vi "CreateScanPattern.vi"(6 "AO\nrow: rest, illumination\ncol: X, Y, Z":dbl[][](array[numeric])=[[5.0, 5.0, 0.0, 0.0, 0.0, 1.0], [-0.2, 2.9, 0.0, 0.0, 0.0, 0.0]], 8 "Timing":T2={"Size (pix)"=1024, "Exposure (s)"=0.1, "Slice (s)"=0.0, "Series (s)"=0.0} {"Size (pix)" items=["2048"=2048, "1024"=1024, "512"=512, "256"=256]}, 9 "Beam":T5={"n spirals"=5, "A spiral (V)"=0.8, "sigma"=2.0, "SLIM"=TRUE}, 10 "DAQ":T4={"Ramp time (s)"=0.01, "DAQ rate (Hz)"=10000.0, "X0 (V)"=5.0, "Xc (V)"=-0.2, "Y0 (V)"=5.0, "Yc (V)"=-0.2, "Z0 (V)"=0.0, "Zc (V)"=0.0}, 11 "Stack":T3={"LED (V)"=1.0, "#z steps"=1, "z step (V)"=1.0, "UV (%)"=0.2} {"UV (%)" format="%#_13g"}) -> (1 "AO (V)":dbl[][](array[numeric]), 3 "Camera \nExposure Time (ms)":dbl=17.0, 4 "DO":digitaldata[](array[digital]), 5 "All signals":dbl[][](graph))   [LabVIEW 2018]
uses:
  <vilib>/Analysis/1siggen.llb/Ramp Pattern by Samples.vi
  <vilib>/Analysis/baseanly.llb/Mean (DBL).vi
  <vilib>/Analysis/NI_AALBase.lvlib
panel:
  in  "45 Degrees":bool
  in  "A_y":dbl=0.86 format="%#_13g"
  in  "Additional Sweeps/Line":u32=3
  out "fraction exposed":dbl=0.89
  out "Camera\nreadout time (ms)":u64=11
  in  "Channels":T1(ring)=enum."UV"
  out "error out (no error)":errorcluster
  in  "error in (no error)":errorcluster
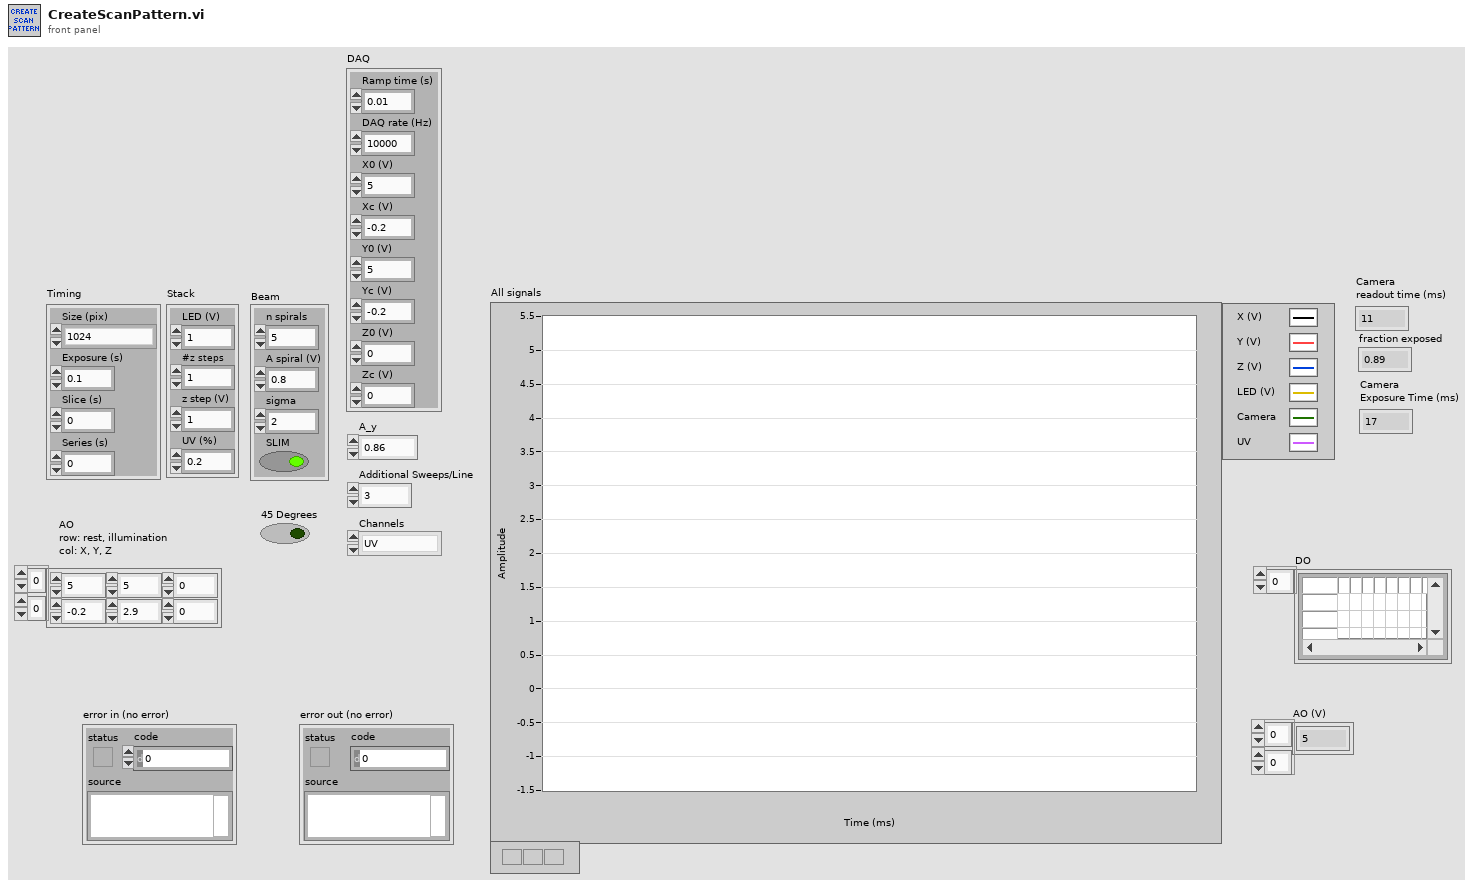
[diagram p1: front panel]
types:
  T1 = enum16{"X (V)", "Y (V)", "Z (V)", "LED (V)", "Camera", "UV"}
  T2 = cluster{"Size (pix)":u16, "Exposure (s)":dbl, "Slice (s)":dbl, "Series (s)":dbl}
  T3 = cluster{"LED (V)":dbl, "#z steps":i64, "z step (V)":dbl, "UV (%)":dbl}
  T4 = cluster{"Ramp time (s)":dbl, "DAQ rate (Hz)":dbl, "X0 (V)":dbl, "Xc (V)":dbl, "Y0 (V)":dbl, "Yc (V)":dbl, "Z0 (V)":dbl, "Zc (V)":dbl}
  T5 = cluster{"n spirals":u32, "A spiral (V)":dbl, "sigma":dbl, "SLIM":bool}
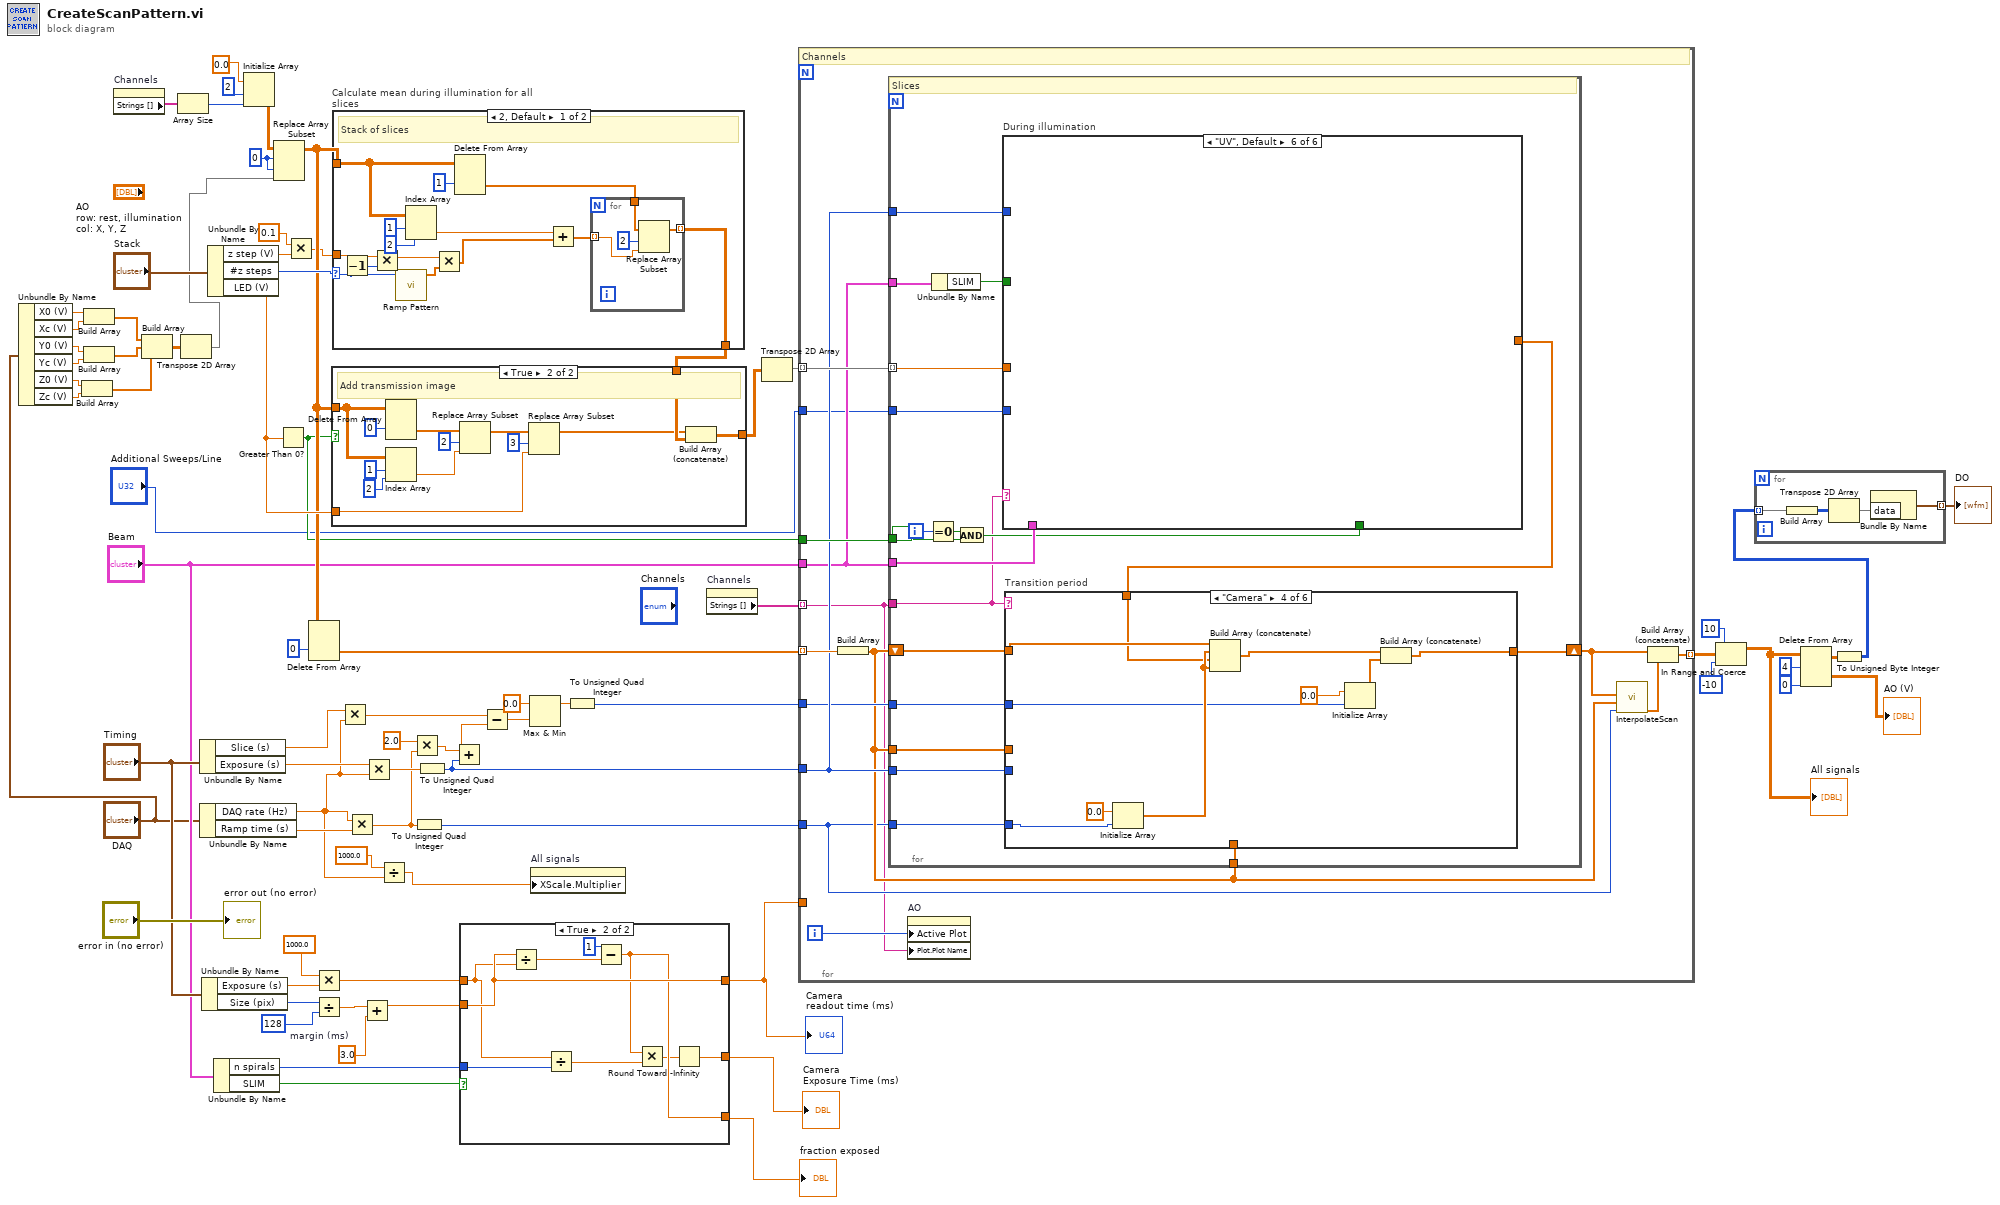
[diagram p0: block diagram]
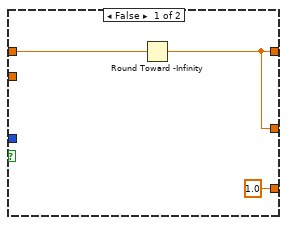
[diagram p2: hidden frame]
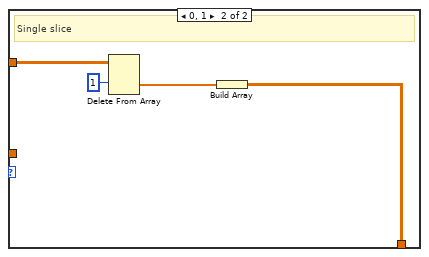
[diagram p4: hidden frame]
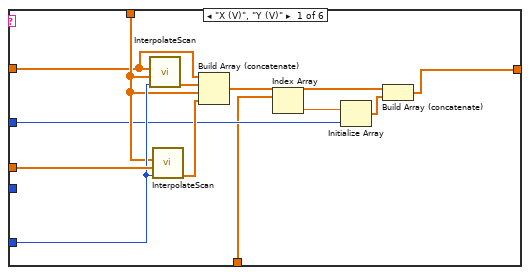
[diagram p5: hidden frame]
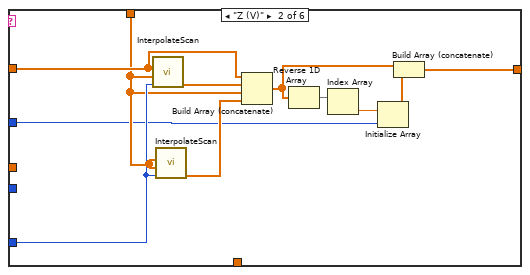
[diagram p6: hidden frame]
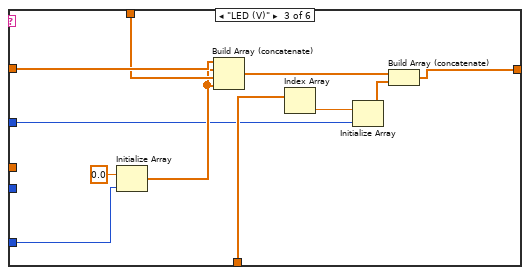
[diagram p7: hidden frame]
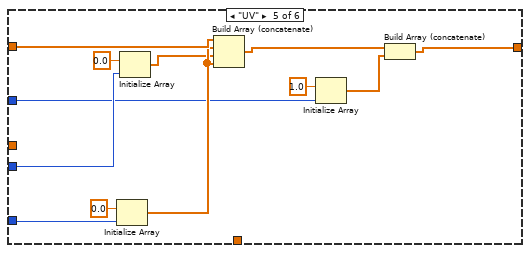
[diagram p8: hidden frame]
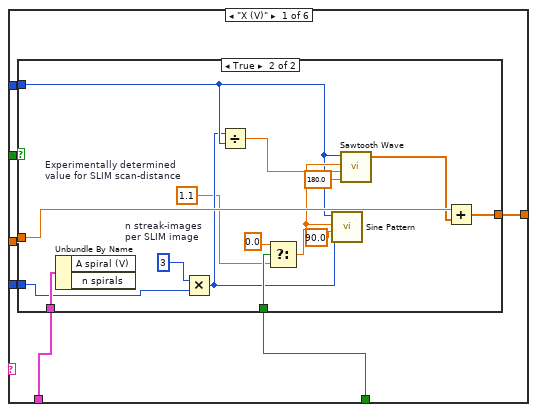
[diagram p10: hidden frame]
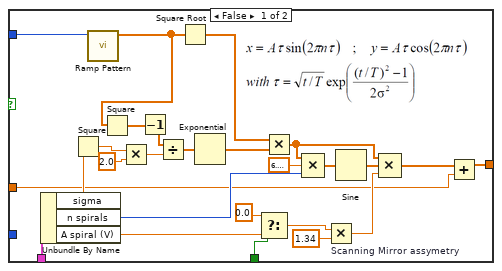
[diagram p11: hidden frame]
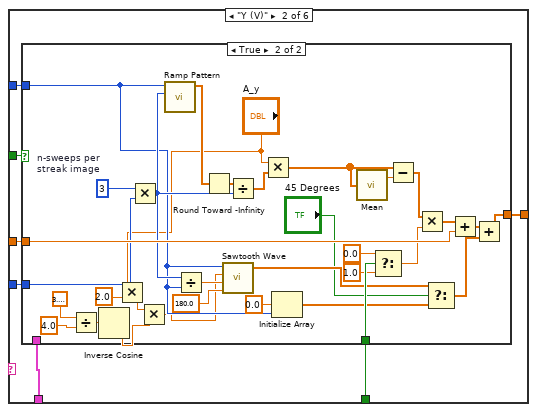
[diagram p12: hidden frame]
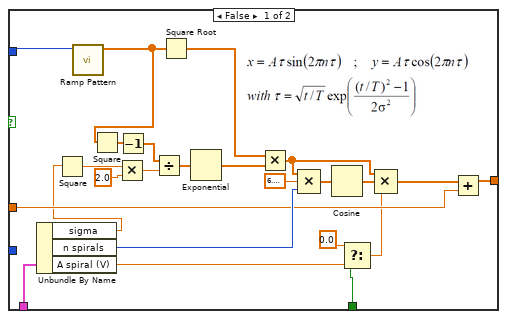
[diagram p13: hidden frame]
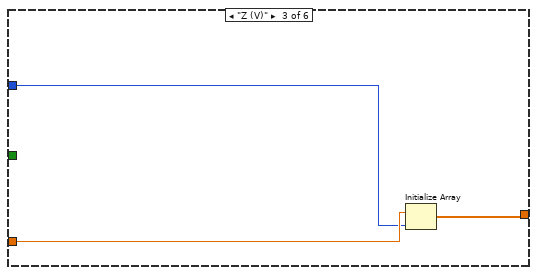
[diagram p14: hidden frame]
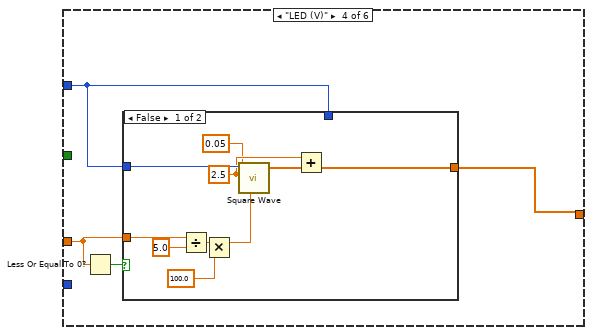
[diagram p15: hidden frame]
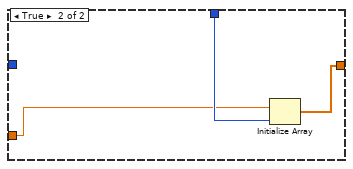
[diagram p16: hidden frame]
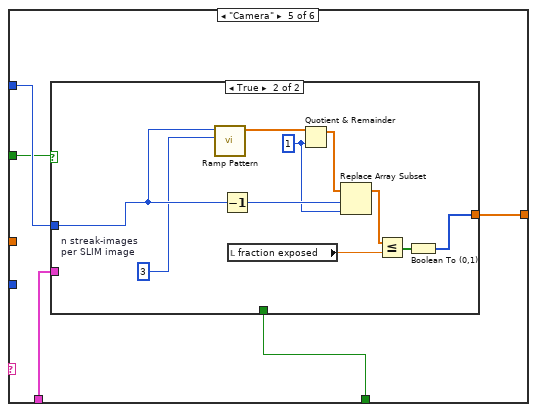
[diagram p17: hidden frame]
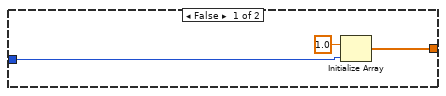
[diagram p18: hidden frame]
diagram:
  w27 = 3.0  # margin (ms)
  w63 = 0 ("index (row)")
  n1 = Unbundle By Name("DAQ") -> ("X0 (V)"=w11:dbl, "Xc (V)"=w10:dbl, "Y0 (V)"=w9:dbl, "Yc (V)"=w8:dbl, "Z0 (V)"=w6:dbl, "Zc (V)"=w7:dbl)
  n2 = Build Array(w6, w7) -> (w3:dbl[])
  n3 = Build Array(w11, w10) -> (w5:dbl[])
  n4 = Build Array(w9, w8) -> (w4:dbl[])
  n5 = property on="Channels" class="Enum (strict)"() -> ("Strings []"=w54:string[])  [unwired: 2 in, 2 out]
  n6 = Build Array(w5, w4, w3) -> (w2:dbl[][])
  n7 = Array Size(array=w54) -> (size(s)=w53:i32)
  n8 = Transpose 2D Array(2D array=w2) -> (transposed array=w1:dbl[][])
  n9 = Unbundle By Name("Timing") -> ("Slice (s)"=w61:dbl, "Exposure (s)"=w77:dbl)
  n10 = Unbundle By Name("DAQ") -> ("DAQ rate (Hz)"=w32:dbl, "Ramp time (s)"=w71:dbl)
  n11 = Unbundle By Name("Timing") -> ("Exposure (s)"=w34:dbl, "Size (pix)"=w40:u16)
  n12 = Unbundle By Name("Stack") -> ("z step (V)"=w17:dbl, "#z steps"=w72:i64, "LED (V)"=w68:dbl)
  n13 = Unbundle By Name("Beam") -> ("n spirals"=w36:u32, "SLIM"=w38:bool)
  n14 = Initialize Array(0.0 ("dimension size"), 2 ("dimension size"), w53) -> (w64:dbl[][])
  n15 = Replace Array Subset(array=w64, new element=w1, index (row)=w63, index (col)=w63) -> (w62:dbl[][])
  n16 = Greater Than 0?(x=w68) -> (x > 0?=w52:bool)
  n17 = Multiply(x=0.1, y=w17) -> (x*y=w18:dbl)
  n18 = Delete From Array(array=w62, index (row)=0) -> (deleted portion=w13:dbl[])  [unwired: 2 in, 1 out]
  n19 = Multiply(x=1000.0 ("y"), y=w34) -> (x*y=w33:dbl)
  n20 = Divide(x=w40, y=u16 128) -> (x/y=w37:dbl)
  n21 = case "Calculate mean during illumination for all slices" shown="2, Default" w72 {
    selector: w72 -> [w80 _]
    tunnel: w62 -> [w84 w98]
    tunnel: w18 -> [w90 _]
    tunnel: [w83 w97] -> w70
    frame 2, Default {
      # "Stack of slices"
      n22 = Decrement(x=w80) -> (x-1=w79:i64)
      n23 = Multiply(x=w90, y=w79) -> (x*y=w81:dbl)
      n24 = call-poly <vilib>:"Ramp Pattern.vi"("samples"=w80) -> ("Ramp Pattern"=w91:dbl[])  [unwired: 9 in, 1 out]
      n25 = Index Array(array=w84, index (row)=1, index (col)=2 ("disabled index (col)")) -> (element=w87:dbl)
      n26 = Multiply(x=w81, y=w91) -> (x*y=w78:dbl[])
      n27 = Delete From Array(array=w84, index (row)=1) -> (deleted portion=w82:dbl[])  [unwired: 2 in, 1 out]
      n28 = Add(x=w87, y=w78) -> (x+y=w86:dbl[])
      n29 = for {
        tunnel: w86 -> [w93] mode=indexing
        tunnel: w82 -> [w95]
        tunnel: [w92] -> w83 mode=indexing
        n30 = Replace Array Subset(array=w95, new element=w93, index=2) -> (w92:dbl[])
      }
    }
    frame 0, 1 {
      # "Single slice"
      n31 = Delete From Array(array=w98, index (row)=1) -> (deleted portion=w96:dbl[])  [unwired: 2 in, 1 out]
      n32 = Build Array(w96) -> (w97:dbl[][])
    }
  }
  n33 = case shown="True" w52 {
    tunnel: [w100 w105] -> w69
    tunnel: w70 -> [w100 w106]
    tunnel: w62 -> [_ w110]
    tunnel: w68 -> [_ w101]
    frame False {
      # "No transmission image"
    }
    frame True {
      # "Add transmission image"
      n34 = Delete From Array(array=w110, index (row)=0) -> (deleted portion=w112:dbl[])  [unwired: 2 in, 1 out]
      n35 = Index Array(array=w110, index (row)=1, index (col)=2 ("disabled index (col)")) -> (element=w107:dbl)
      n36 = Replace Array Subset(array=w112, new element=w107, index=2) -> (w103:dbl[])
      n37 = Replace Array Subset(array=w103, new element=w101, index=3) -> (w104:dbl[])
      n38 = Build Array (concatenate)(w104, w106) -> (w105:dbl[][])
    }
  }
  n39 = Multiply(x=w61, y=w32) -> (x*y=w56:dbl)
  n40 = Multiply(x=w32, y=w71) -> (x*y=w60:dbl)
  n41 = Add(x=w37, y=w27) -> (x+y=w28:dbl)
  n42 = Multiply(x=w77, y=w32) -> (x*y=w73:dbl)
  n43 = Divide(x=1000.0, y=w32) -> (x/y=w29:dbl)
  n44 = Multiply(x=2.0, y=w60) -> (x*y=w58:dbl)
  n45 = To Unsigned Quad Integer(1:w60) -> (0:w50:u64)
  n46 = To Unsigned Quad Integer(1:w73) -> (0:w48:u64)
  n47 = Add(x=w58, y=w48) -> (x+y=w57:dbl)
  n48 = case shown="True" w38 {
    tunnel: w28 -> [_ w123]
    tunnel: w36 -> [_ w121]
    tunnel: [w114 w123] -> w15
    tunnel: w33 -> [w115 w122]
    tunnel: [1.0 w119] -> w30
    tunnel: [w114 w117] -> w19
    frame False {
      n49 = Round Toward -Infinity(1:w115) -> (0:w114:dbl)
    }
    frame True {
      n50 = Divide(x=w123, y=w122) -> (x/y=w125:dbl)
      n51 = Divide(x=w122, y=w121) -> (x/y=w120:dbl)
      n52 = Subtract(x=1 ("index (row)"), y=w125) -> (x-y=w119:dbl)
      n53 = Multiply(x=w119, y=w120) -> (x*y=w118:dbl)
      n54 = Round Toward -Infinity(1:w118) -> (0:w117:dbl)
    }
  }
  "Camera\nreadout time (ms)" <- w15
  "fraction exposed" <- w30
  "Camera \nExposure Time (ms)" <- w19
  n55 = Subtract(x=w56, y=w57) -> (x-y=w55:dbl)
  n56 = Max & Min(x=0.0, y=w55) -> (max(x,y)=w47:dbl)  [unwired: 1 out]
  n57 = property on="All signals" class="WFGraph (strict)"("XScale.Multiplier"=w29) -> ()  [unwired: 2 in, 2 out]
  n58 = To Unsigned Quad Integer(1:w47) -> (0:w49:u64)
  n59 = property on="Channels" class="Enum (strict)"() -> ("Strings []"=w75:string[])  [unwired: 2 in, 2 out]
  n60 = Transpose 2D Array(2D array=w69) -> (transposed array=w51:dbl[][])
  n61 = for {
    tunnel: w75 -> [w129] mode=indexing
    tunnel: "Beam" -> [w128]
    tunnel: w51 -> [w139] mode=indexing
    tunnel: w13 -> [w137] mode=indexing
    tunnel: w50 -> [w131]
    tunnel: w49 -> [w133]
    tunnel: w52 -> [w138]
    tunnel: w48 -> [w134]
    tunnel: [w127] -> w24 mode=indexing
    tunnel: w15 -> [_]
    tunnel: "Additional Sweeps/Line" -> [w126]
    i -> [w130]
    # "Channels"
    n62 = Build Array(w137) -> (w132:dbl[])
    n63 = for {
      tunnel: w129 -> [w150]
      tunnel: w128 -> [w158]
      tunnel: w139 -> [w157] mode=indexing
      tunnel: w138 -> [w154]
      tunnel: w134 -> [w152]
      shift-right: [w147] -> w135
      shift-left: w132 -> [w149]
      tunnel: w131 -> [w148]
      tunnel: w132 -> [w146]
      tunnel: w134 -> [w145]
      tunnel: w133 -> [w144]
      tunnel: w132 -> [w143]
      tunnel: w128 -> [w142]
      tunnel: w126 -> [w140]
      i -> [w156]
      # "Slices"
      n64 = Equal To 0?(x=w156) -> (x = 0?=w155:bool)
      n65 = Unbundle By Name(w142) -> ("SLIM"=w141:bool)
      n66 = And(x=w155, y=w154) -> (x .and. y?=w153:bool)
      n67 = case "During illumination" shown="\"UV\", Default" w150 {
        tunnel: w158 -> [w221 w269 _ _ w348 _]
        tunnel: [w220 w268 w329 w333 w351 _] -> w151
        tunnel: w157 -> [w219 w267 w328 w331 _ _]
        tunnel: w153 -> [w218 w266 _ _ w347 _]
        tunnel: w152 -> [w216 w264 w327 w332 w350 _]
        tunnel: w141 -> [w217 w265 _ _ w349 _]
        tunnel: w140 -> [w215 w263 _ _ _ _]
        frame "X (V)" {
          n68 = case shown="True" w217 {
            tunnel: w221 -> [w233 w262]
            tunnel: [w232 w261] -> w220
            tunnel: w219 -> [w231 w257]
            tunnel: w218 -> [w227 w259]
            tunnel: w216 -> [w224 w253]
            tunnel: w215 -> [_ w256]
            frame False {
              n69 = Unbundle By Name(w233) -> ("sigma"=w236:dbl, "n spirals"=w237:u32, "A spiral (V)"=w229:dbl)
              n70 = Square(x=w236) -> (x^2=w247:dbl)
              n71 = call-poly <vilib>:"Ramp Pattern.vi"("samples"=w224) -> ("Ramp Pattern"=w223:dbl[])  [unwired: 9 in, 1 out]
              n72 = Square(x=w223) -> (x^2=w225:dbl[])
              n73 = Multiply(x=w247, y=2.0) -> (x*y=w245:dbl)
              n74 = Decrement(x=w225) -> (x-1=w226:dbl[])
              n75 = Divide(x=w226, y=w245) -> (x/y=w244:dbl[])
              n76 = Square Root(x=w223) -> (sqrt(x)=w243:dbl[])
              n77 = Exponential(1:w244) -> (0:w242:dbl[])
              n78 = Select(t=0.0 ("f"), s=w227, f=w229) -> (s? t:f=w228:dbl)
              n79 = Multiply(x=w243, y=w242) -> (x*y=w239:dbl[])
              n80 = Compound Arithmetic op=MULTIPLY(w239, 6.283185307179586, w237) -> (w238:dbl[])
              n81 = Multiply "Scanning Mirror assymetry"(x=w228, y=1.34 ("x")) -> (x*y=w234:dbl)
              n82 = Sine(x=w238) -> (sin(x)=w240:dbl[])
              n83 = Compound Arithmetic op=MULTIPLY(w239, w240, w234) -> (w222:dbl[])
              n84 = Add(x=w222, y=w231) -> (x+y=w232:dbl[])
            }
            frame True {
              w248 = u32 3  # n streak-images  per SLIM image
              w249 = 1.1  # Experimentally determined  value for SLIM scan-distance
              n85 = Unbundle By Name(w262) -> ()  [unwired: 2 out]
              n86 = Multiply(x=w248, y=w256) -> (x*y=w252:u32)
              n87 = Divide(x=w252, y=w253) -> (x/y=w251:dbl)
              n88 = Select(t=0.0 ("f"), s=w259, f=w249) -> (s? t:f=w255:dbl)
              n89 = call <vilib>:"Sine Pattern.vi"("cycles"=w252, "phase(degrees)"=90.0, "amplitude"=w255, "samples"=w253) -> ()  [unwired: 2 out]
              n90 = call <vilib>:"Sawtooth Wave.vi"("samples"=w253, "amplitude"=w255, "frequency"=w251, "phase in"=180.0) -> ("sawtooth wave"=w254:dbl[])  [unwired: 1 in, 2 out]
              n91 = Add(x=w257, y=w254) -> (x+y=w261:dbl[])
            }
          }
        }
        frame "Y (V)" {
          n92 = case shown="True" w265 {
            tunnel: w269 -> [w281 _]
            tunnel: [w280 w300] -> w268
            tunnel: w267 -> [w279 w326]
            tunnel: w266 -> [w275 w325]
            tunnel: w264 -> [w273 w309]
            tunnel: w263 -> [_ w318]
            frame False {
              n93 = Unbundle By Name(w281) -> ("sigma"=w271:dbl, "n spirals"=w282:u32, "A spiral (V)"=w278:dbl)
              n94 = Square(x=w271) -> (x^2=w292:dbl)
              n95 = call-poly <vilib>:"Ramp Pattern.vi"("samples"=w273) -> ("Ramp Pattern"=w272:dbl[])  [unwired: 9 in, 1 out]
              n96 = Square(x=w272) -> (x^2=w293:dbl[])
              n97 = Multiply(x=w292, y=2.0) -> (x*y=w290:dbl)
              n98 = Decrement(x=w293) -> (x-1=w274:dbl[])
              n99 = Divide(x=w274, y=w290) -> (x/y=w289:dbl[])
              n100 = Square Root(x=w272) -> (sqrt(x)=w288:dbl[])
              n101 = Exponential(1:w289) -> (0:w287:dbl[])
              n102 = Multiply(x=w288, y=w287) -> (x*y=w284:dbl[])
              n103 = Compound Arithmetic op=MULTIPLY(w284, 6.283185307179586, w282) -> (w283:dbl[])
              n104 = Cosine(x=w283) -> (cos(x)=w285:dbl[])
              n105 = Select(t=0.0 ("f"), s=w275, f=w278) -> (s? t:f=w276:dbl)
              n106 = Compound Arithmetic op=MULTIPLY(w284, w285, w276) -> (w270:dbl[])
              n107 = Add(x=w270, y=w279) -> (x+y=w280:dbl[])
            }
            frame True {
              w294 = u32 3  # n-sweeps per streak image
              n108 = Divide(x=3.141592653589793, y=4.0) -> (x/y=w312:dbl)
              n109 = Inverse Cosine(1:w312) -> (0:w299:dbl)
              n110 = Multiply(x="A_y", y=2.0) -> (x*y=w297:dbl)
              n111 = Multiply(x=w294, y=w318) -> (x*y=w317:u32)
              n112 = Multiply(x=w297, y=w299) -> (x*y=w298:dbl)
              n113 = call-poly <vilib>:"Ramp Pattern.vi"("end"=w317, "samples"=w309) -> ("Ramp Pattern"=w305:dbl[])  [unwired: 8 in, 1 out]
              n114 = Divide(x=w317, y=w309) -> (x/y=w316:dbl)
              n115 = Round Toward -Infinity(1:w305) -> (0:w319:dbl[])
              n116 = call <vilib>:"Sawtooth Wave.vi"("samples"=w309, "amplitude"=w298, "frequency"=w316, "phase in"=180.0) -> ("sawtooth wave"=w311:dbl[])  [unwired: 1 in, 2 out]
              n117 = Divide(x=w319, y=w317) -> (x/y=w324:dbl[])
              n118 = Multiply(x="A_y", y=w324) -> (x*y=w306:dbl[])
              n119 = Initialize Array(0.0 ("element"), w309) -> (w308:dbl[])
              n120 = call-poly <vilib>:"Mean.vi"("X"=w306) -> ("mean"=w323:dbl)  [unwired: 1 out]
              n121 = Select(t=0.0 ("f"), s=w325, f=1.0) -> (s? t:f=w320:dbl)
              n122 = Subtract(x=w306, y=w323) -> (x-y=w304:dbl[])
              n123 = Multiply(x=w304, y=w320) -> (x*y=w303:dbl[])
              n124 = Select(t=w311, s="45 Degrees", f=w308) -> (s? t:f=w301:dbl[])
              n125 = Add(x=w303, y=w326) -> (x+y=w302:dbl[])
              n126 = Add(x=w302, y=w301) -> (x+y=w300:dbl[])
            }
          }
        }
        frame "Z (V)" {
          n127 = Initialize Array(w328, w327) -> (w329:dbl[])
        }
        frame "LED (V)" {
          n128 = Less Or Equal To 0?(x=w331) -> (x <= 0?=w330:bool)
          n129 = case shown="False" w330 {
            tunnel: w331 -> [w343 w344]
            tunnel: w332 -> [w340 _]
            tunnel: [w339 w345] -> w333
            tunnel: w332 -> [_ w346]
            frame False {
              w338 = 2.5 ("amplitude")
              n130 = Divide(x=w343, y=5.0) -> (x/y=w342:dbl)
              n131 = Multiply(x=w342, y=100.0) -> (x*y=w335:dbl)
              n132 = call <vilib>:"Square Wave.vi"("samples"=w340, "amplitude"=w338, "frequency"=0.05, "duty cycle (%)"=w335) -> ("square wave"=w336:dbl[])  [unwired: 2 in, 2 out]
              n133 = Add(x=w338, y=w336) -> (x+y=w339:dbl[])
            }
            frame True {
              n134 = Initialize Array(w344, w346) -> (w345:dbl[])
            }
          }
        }
        frame "Camera" {
          n135 = case shown="True" w349 {
            tunnel: [w354 w361] -> w351
            tunnel: w350 -> [w352 w356]
            tunnel: w348 -> [_ _]
            tunnel: w347 -> [_ _]
            frame False {
              n136 = Initialize Array(1.0 ("element"), w352) -> (w354:dbl[])
            }
            frame True {
              w355 = u32 3  # n streak-images  per SLIM image
              w357 = 1 ("index")
              n137 = call-poly <vilib>:"Ramp Pattern.vi"("end"=w355, "samples"=w356) -> ("Ramp Pattern"=w362:dbl[])  [unwired: 8 in, 1 out]
              n138 = Decrement(x=w356) -> (x-1=w359:u64)
              n139 = local read "fraction exposed"() -> (w363:dbl)
              n140 = Quotient & Remainder(x=w362, y=w357) -> (x-y*floor(x/y)=w360:dbl[])  [unwired: 1 out]
              n141 = Replace Array Subset(array=w360, new element=w357, index=w359) -> (w358:dbl[])
              n142 = Less Or Equal?(x=w358, y=w363) -> (x <= y?=w364:bool[])
              n143 = Boolean To (0,1)(Boolean=w364) -> (0, 1=w361:i16[])
            }
          }
        }
        frame "UV", Default {
        }
      }
      n144 = case "Transition period" shown="\"Camera\"" w150 {
        tunnel: w151 -> [w167 w177 w189 w194 _ _]
        tunnel: w149 -> [w165 w178 w190 w201 w212 _]
        tunnel: w146 -> [w170 _ _ _ _ _]
        tunnel: w148 -> [w169 w181 w192 w193 w214 _]
        tunnel: [w163 w176 w186 w198 w206 _] -> w147
        tunnel: w145 -> [_ _ _ _ w209 _]
        tunnel: w144 -> [w162 w174 w183 w197 w205 _]
        tunnel: w143 -> [w161 _ w184 _ _ _]
        frame "X (V)", "Y (V)" {
          n145 = call "InterpolateScan.vi"("samples"=w169, "end"=w167, "start"=w165) -> ("interpolated"=w168:dbl[])  [unwired: 8 in]
          n146 = call "InterpolateScan.vi"("samples"=w169, "end"=w170, "start"=w167) -> ("interpolated"=w166:dbl[])  [unwired: 8 in]
          n147 = Build Array (concatenate)(w165, w168, w167, w166) -> (w164:dbl[])
          n148 = Index Array(array=w161) -> (element=w160:dbl)  [unwired: 1 in]
          n149 = Initialize Array(w160, w162) -> (w159:dbl[])
          n150 = Build Array (concatenate)(w164, w159) -> (w163:dbl[])
        }
        frame "Z (V)" {
          n151 = call "InterpolateScan.vi"("samples"=w181, "end"=w177, "start"=w178) -> ("interpolated"=w180:dbl[])  [unwired: 8 in]
          n152 = call "InterpolateScan.vi"("samples"=w181, "end"=w177, "start"=w177) -> ("interpolated"=w179:dbl[])  [unwired: 8 in]
          n153 = Build Array (concatenate)(w178, w180, w177, w179) -> (w172:dbl[])
          n154 = Reverse 1D Array(array=w172) -> (reversed array=w171:dbl[])
          n155 = Index Array(array=w171) -> (element=w175:dbl)  [unwired: 1 in]
          n156 = Initialize Array(w175, w174) -> (w173:dbl[])
          n157 = Build Array (concatenate)(w172, w173) -> (w176:dbl[])
        }
        frame "LED (V)" {
          n158 = Initialize Array(0.0 ("element"), w192) -> (w188:dbl[])
          n159 = Build Array (concatenate)(w190, w188, w189, w188) -> (w187:dbl[])
          n160 = Index Array(array=w184) -> (element=w185:dbl)  [unwired: 1 in]
          n161 = Initialize Array(w185, w183) -> (w182:dbl[])
          n162 = Build Array (concatenate)(w187, w182) -> (w186:dbl[])
        }
        frame "Camera" {
          n163 = Initialize Array(0.0 ("element"), w193) -> (w200:dbl[])
          n164 = Build Array (concatenate)(w201, w200, w194, w200) -> (w199:dbl[])
          n165 = Initialize Array(0.0 ("element"), w197) -> (w195:dbl[])
          n166 = Build Array (concatenate)(w199, w195) -> (w198:dbl[])
        }
        frame "UV" {
          n167 = Initialize Array(0.0 ("element"), w214) -> (w211:dbl[])
          n168 = Initialize Array(0.0 ("element"), w209) -> (w208:dbl[])
          n169 = Build Array (concatenate)(w212, w211, w208, w211) -> (w207:dbl[])
          n170 = Initialize Array(1.0 ("element"), w205) -> (w203:dbl[])
          n171 = Build Array (concatenate)(w207, w203) -> (w206:dbl[])
        }
        frame "False", Default {
        }
      }
    }
    n172 = property on="AO" class="WFGraph (strict)"("Active Plot"=w130, "Plot.Plot Name"=w129) -> ()  [unwired: 2 in, 2 out]
    n173 = call "InterpolateScan.vi"("samples"=w131, "end"=w132, "start"=w135) -> ("interpolated"=w136:dbl[])  [unwired: 8 in]
    n174 = Build Array (concatenate)(w135, w136) -> (w127:dbl[])
  }
  n175 = In Range and Coerce(upper limit=10, x=w24, lower limit=-10) -> (coerced(x)=w21:dbl[][])  [unwired: 1 out]
  "All signals" <- w21
  n176 = Delete From Array(array=w21, length=4, index (row)=0) -> (deleted portion=→"AO (V)":dbl[][], array with subset deleted=w44:dbl[][])  [unwired: 1 in]
  n177 = To Unsigned Byte Integer(number=w44) -> (unsigned 8bit integer=w26:u8[][])
  n178 = for {
    tunnel: [w368] -> w25 mode=indexing
    tunnel: w26 -> [w365] mode=indexing
    n179 = Build Array(w365) -> (w367:u8[][])
    n180 = Transpose 2D Array(2D array=w367) -> (transposed array=w366:u8[][])
    n181 = Bundle By Name("data"=w366) -> (w368:digitaldata)  [unwired: 1 in]
  }
  "DO" <- w25
  "error out (no error)" <- "error in (no error)"
